vi "test_write_AB2504_2.vi"() -> ()   [LabVIEW 2015, in "Tausand AB1000.lvlib"]
uses:
  <instrlib>/Tausand AB1000/Tausand AB1000.lvlib
  <instrlib>/Tausand AB1000/Public/Controls/configMultipleCoincRing.ctl
  <instrlib>/Tausand AB1000/Public/Controls/channelRing.ctl
  <instrlib>/Tausand AB1000/Public/Controls/deviceTypeRing.ctl
panel:
  out "error?":bool
  in  "channel 2":T1 items=["none", "A", "B", "C", "D", "E", "F", "G", "H"]
  in  "delay Ch2 (0 ns)":u32 step=2
  in  "delay Ch1 (0 ns)":u32 step=2
  in  "channel 1":T1 items=["none", "A", "B", "C", "D", "E", "F", "G", "H"]
  in  "Multiple coincidence configuration":T2=240 caption="multi-fold chan. (xF0: ABCD)" format="%b" items=["ABC"=224, "ABD"=208, "ABE"=200, "ABF"=196, "ABG"=194, "ABH"=193, "ACD"=176, "ACE"=168, "ACF"=164, "ACG"=162, "ACH"=161, "ADE"=152, "ADF"=148, "ADG"=146, "ADH"=145, "AEF"=140, "AEG"=138, "AEH"=137, "AFG"=134, "AFH"=133, "AGH"=131, "BCD"=112, "BCE"=104, "BCF"=100, "BCG"=98, "BCH"=97, "BDE"=88, "BDF"=84, "BDG"=82, "BDH"=81, "BEF"=76, "BEG"=74, "BEH"=73, "BFG"=70, "BFH"=69, "BGH"=67, "CDE"=56, "CDF"=52, "CDG"=50, "CDH"=49, "CEF"=44, "CEG"=42, "CEH"=41, "CFG"=38, "CFH"=37, "CGH"=35, "DEF"=28, "DEG"=26, "DEH"=25, "DFG"=22, "DFH"=21, "DGH"=19, "EFG"=14, "EFH"=13, "EGH"=11, "FGH"=7, "ABCD"=240, "ABCE"=232, "ABCF"=228, "ABCG"=226, "ABCH"=225, "ABDE"=216, "ABDF"=212, "ABDG"=210, "ABDH"=209, "ABEF"=204, "ABEG"=202, "ABEH"=201, "ABFG"=198, "ABFH"=197, "ABGH"=195, "ACDE"=184, "ACDF"=180, "ACDG"=178, "ACDH"=177, "ACEF"=172, "ACEG"=170, "ACEH"=169, "ACFG"=166, "ACFH"=165, "ACGH"=163, "ADEF"=156, "ADEG"=154, "ADEH"=153, "ADFG"=150, "ADFH"=149, "ADGH"=147, "AEFG"=142, "AEFH"=141, "AEGH"=139, "AFGH"=135, "BCDE"=120, "BCDF"=116, "BCDG"=114, "BCDH"=113, "BCEF"=108, "BCEG"=106, "BCEH"=105, "BCFG"=102, "BCFH"=101, "BCGH"=99, "BDEF"=92, "BDEG"=90, "BDEH"=89, "BDFG"=86, "BDFH"=85, "BDGH"=83, "BEFG"=78, "BEFH"=77, "BEGH"=75, "BFGH"=71, "CDEF"=60, "CDEG"=58, "CDEH"=57, "CDFG"=54, "CDFH"=53, "CDGH"=51, "CEFG"=46, "CEFH"=45, "CEGH"=43, "CFGH"=39, "DEFG"=30, "DEFH"=29, "DEGH"=27, "DFGH"=23, "EFGH"=15]
  in  "cw value ns (10ns)":u32=10 step=2
  in  "smp value (1000 ms)":u32=1000
  in  "VISA resource name":refnum<visa-resource-name>
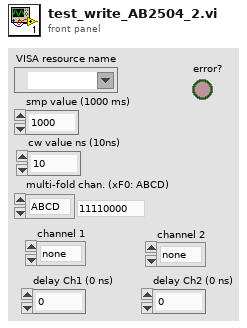
[diagram p1: front panel]
types:
  T1 = typedef "Tausand AB1000.lvlib/channelRing.ctl" = u8
  T2 = typedef "Tausand AB1000.lvlib/configMultipleCoincRing.ctl" = u16
  T3 = typedef "Tausand AB1000.lvlib/deviceTypeRing.ctl" = u16
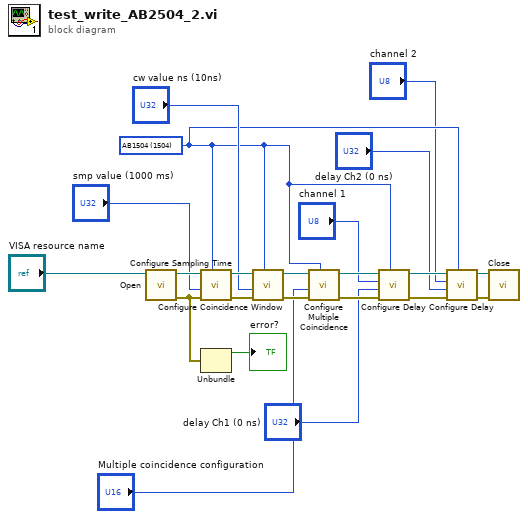
[diagram p0: block diagram]
diagram:
  w11 = T3 1504 items=["any"=0, "AB1002"=1002, "AB1004"=1004, "AB1502"=1502, "AB1504"=1504, "AB1902"=1902, "AB1904"=1904, "AB2002"=2002, "AB2004"=2004, "AB2502"=2502, "AB2504"=2504, "AB2902"=2902, "AB2904"=2904] ("device type")
  n1 = call <instrlib>:"Open.vi"("VISA resource name"="VISA resource name") -> ("error out"=w1:errorcluster, "VISA resource name out"=w22:refnum<visa-resource-name>)  [unwired: 9 in]
  n2 = call <instrlib>:"Configure Sampling Time.vi"("device type"=w11, "error in (no error)"=w1, "value (1000 ms)"="smp value (1000 ms)", "VISA Refnum in"=w22) -> ("error out"=w19:errorcluster, "VISA Refnum out"=w18:refnum<visa-resource-name>)  [unwired: 5 in, 1 out]
  n3 = Unbundle(w1) -> ("status"=→"error?":bool)  [unwired: 2 out]
  n4 = call <instrlib>:"Configure Coincidence Window.vi"("device type"=w11, "error in (no error)"=w19, "value ns (10ns)"="cw value ns (10ns)", "VISA Refnum in"=w18) -> ("error out"=w16:errorcluster, "VISA Refnum out"=w15:refnum<visa-resource-name>)  [unwired: 5 in, 1 out]
  n5 = call <instrlib>:"Configure Multiple Coincidence.vi"("device type"=w11, "error in (no error)"=w16, "Multiple coincidence configuration"="Multiple coincidence configuration", "VISA Refnum in"=w15) -> ("error out"=w10:errorcluster, "VISA Refnum out"=w8:refnum<visa-resource-name>)  [unwired: 6 in]
  n6 = call <instrlib>:"Configure Delay.vi"("device type"=w11, "error in (no error)"=w10, "value (0 ns)"="delay Ch1 (0 ns)", "channel"="channel 1", "VISA Refnum in"=w8) -> ("error out"=w13:errorcluster, "VISA Refnum out"=w12:refnum<visa-resource-name>)  [unwired: 4 in, 1 out]
  n7 = call <instrlib>:"Configure Delay.vi"("device type"=w11, "error in (no error)"=w13, "value (0 ns)"="delay Ch2 (0 ns)", "channel"="channel 2", "VISA Refnum in"=w12) -> ("error out"=w9:errorcluster, "VISA Refnum out"=w7:refnum<visa-resource-name>)  [unwired: 4 in, 1 out]
  n8 = call <instrlib>:"Close.vi"("error in (no error)"=w9, "VISA resource name"=w7) -> ()  [unwired: 9 in, 1 out]
